vi "Communication_Create.vi"(0 "reference in":refnum<class "Communication.lvclass">, 2 "Executer":refnum<class "Executer.lvclass">, 3 "Serializer":refnum<class "Serializer.lvclass">, 5 "error in (no error)":errorcluster) -> (14 "reference out":refnum<class "Communication.lvclass">, 19 "error out":errorcluster)   [LabVIEW 2018, in "Communication.lvclass"]
uses:
  Communication.lvclass
  Executer_class/Executer.lvclass
  Serializers/Serializer_class/Serializer.lvclass
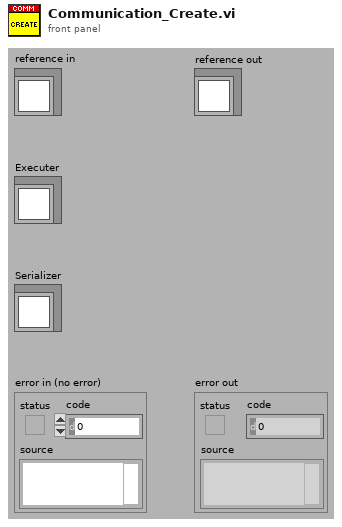
[diagram p1: front panel]
types:
  T1 = typedef "Communication.lvclass/ObjectAttributes.ctl" = cluster{"Executer":refnum<class "Executer.lvclass">, "Serializer":refnum<class "Serializer.lvclass">}
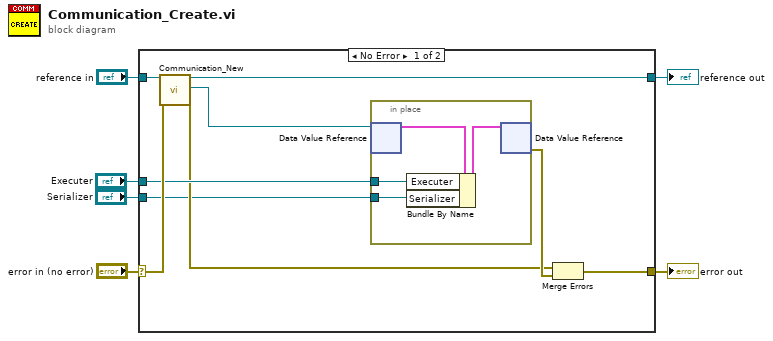
[diagram p0: block diagram]
diagram:
  n1 = case shown="No Error" "error in (no error)" {
    selector: "error in (no error)" -> [w14 w21]
    tunnel: [w11 w21] -> w5
    tunnel: "reference in" -> [w15 w20]
    tunnel: [w13 w20] -> w3
    tunnel: "Executer" -> [w9 _]
    tunnel: "Serializer" -> [w7 _]
    frame No Error {
      n2 = call "Communication_New.vi"("reference in"=w15, "error in (no error)"=w14) -> ("reference out"=w13:refnum<class "Communication.lvclass">, "DVRRefOut"=w10:refnum<data-value>, "error out"=w8:errorcluster)  [unwired: 14 in, 1 out]
      n3 = in-place {
        in-place-border: w9 -> [w17]
        in-place-border: w7 -> [w16]
        n4 = in-place-dvr #1(w10) -> (w18:T1)  [unwired: 1 out]
        n5 = Bundle By Name(cluster=w18, "Executer"=w17, "Serializer"=w16) -> (w19:T1)
        n6 = in-place-dvr #1(w19) -> (w12:errorcluster)  [unwired: 1 out]
      }
      n7 = Merge Errors(w8, w12) -> (w11:errorcluster)
    }
    frame Error {
      # "VI-TechBaseTemplate_Simple_6x8x6"
    }
  }
  "error out" <- w5
  "reference out" <- w3
